vi "[RT] Finite Acq wRearm.vi"() -> ()   [LabVIEW 2015]
doc: "When a finite acquisition terminates, the FPGA automatically rearms itself for another acquisition. You simply need to call rwfm_Start.vi to perform another finite acquisition."
uses:
  <vilib>/NI/cRIO Wfm/ChannelConfig.ctl
  <vilib>/FPGAPlugInAG/sbRIO-9607/niLvFpga_Open_sbRIO-9607.vi
  <vilib>/rvi/interface/common/dynamic/niFpgaDynamicAddResources.vi
  <vilib>/FPGAPlugInAG/Dynamic/niLvFpga_Reset_Dynamic.vi
  <vilib>/FPGAPlugInAG/Dynamic/niLvFpga_Run_Dynamic.vi
  <vilib>/FPGAPlugInAG/Dynamic/niLvFpga_Close_Dynamic.vi
  <vilib>/rvi/interface/nirviOpenFPGA/nirviOpenFPGA.xnode
  FPGA Bitfiles/WaveformLibraryI_FPGATarget2_[FPGA]SARAcqMain_U+qOsuK4w1s.lvbitx
  FPGA/[FPGA] SAR Acq Main.vi
  <vilib>/rvi/interface/nirviMethod/nirviMethod.xnode
  <vilib>/rvi/interface/nirviCloseFPGA/nirviCloseFPGA.xnode
  IFw_Addon/RT/WaveformTask.lvclass
  <vilib>/NI/cRIO Wfm/cRIO Wfm.lvlib
panel:
  in  "Sample Rate":u32=51200
  in  "Channel Info":T1=[{"Channel Name"="Mod1/ai0", "Sensitivity mV_EU"=1000.0, "EU"="V", "dB Ref EU"=1.0}, {"Channel Name"="Mod1/ai1", "Sensitivity mV_EU"=1000.0, "EU"="V", "dB Ref EU"=1.0}, {"Channel Name"="Mod1/ai2", "Sensitivity mV_EU"=1000.0, "EU"="V", "dB Ref EU"=1.0}] caption="Channel Name      Scale [mV/EU]        EU           dB Ref [EU]" {"dB Ref EU" format="%#.2p"; "Sensitivity mV_EU" format="%.2f"}
  in  "Samps per Chan":i32=25600 caption="Samples per Channel"
  in  "stop":bool
  out "Waveform Graph":sgl[][](graph)
  in  "Snapshot":bool
  # "Sampling Info"
  # "Channel Info"
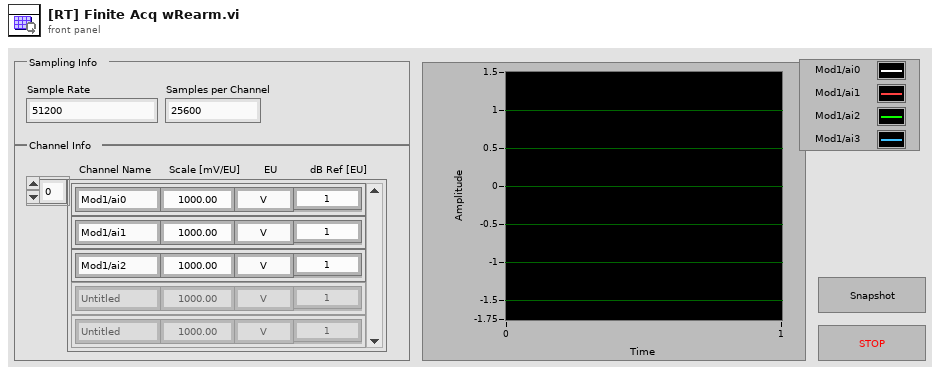
[diagram p1: front panel]
types:
  T1 = typedef "cRIO Wfm.lvlib/ChannelConfig.ctl" = cluster{"Channel Name":string, "Sensitivity mV_EU":dbl, "EU":string, "dB Ref EU":dbl}[]
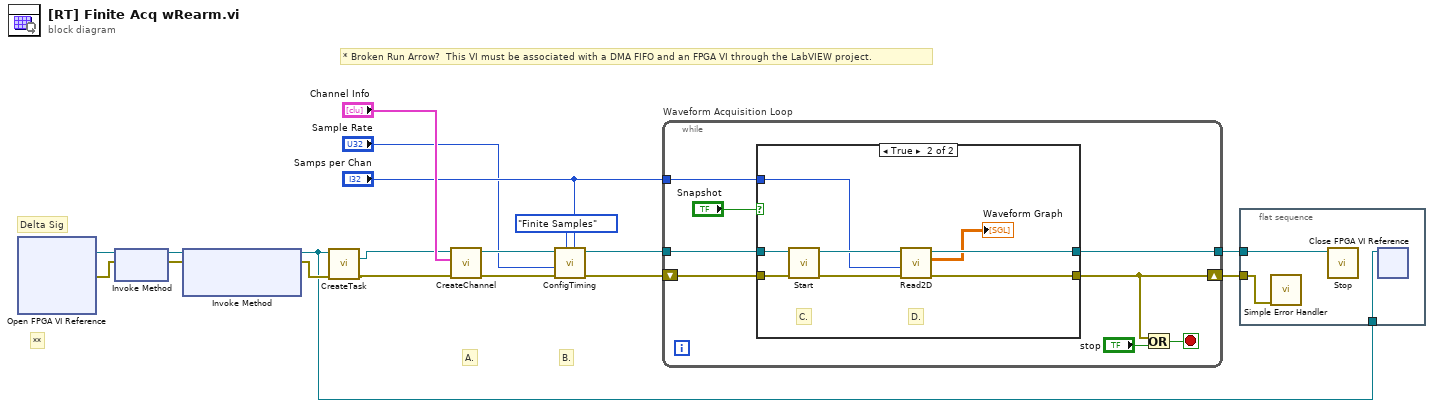
[diagram p0: block diagram]
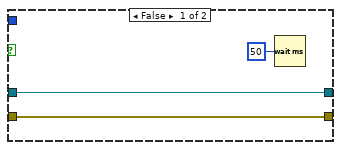
[diagram p2: hidden frame]
diagram:
  # "Delta Sig"
  # "**"
  # "* Broken Run Arrow?  This VI must be associated with a DMA FIFO and an FPGA VI through the LabVIEW project."
  # "B."
  # "A."
  n1 = xnode "Open FPGA VI Reference"() -> ("FPGA VI Reference Out"=w8:refnum<k20>, "error out"=w7:errorcluster)  [unwired: 2 in]
  n2 = xnode "Invoke Method"("FPGA VI Reference In"=w8, "error in"=w7) -> ("FPGA VI Reference Out"=w10:refnum<k20>, "error out"=w9:errorcluster)
  n3 = xnode "Invoke Method"("FPGA VI Reference In"=w10, "error in"=w9) -> ("FPGA VI Reference Out"=w2:refnum<k20>, "error out"=w6:errorcluster)  [unwired: 1 in]
  n4 = call "CreateTask.vi"("FPGA Ref in"=w2, "error in"=w6) -> ("Task out"=w5:refnum<class "WaveformTask.lvclass">, "error out"=w4:errorcluster)  [unwired: 11 in, 1 out]
  n5 = call "CreateChannel.vi"("error in"=w4, "Channel Info"="Channel Info", "task in"=w5) -> ("error out"=w14:errorcluster, "Task out"=w15:refnum<class "WaveformTask.lvclass">)  [unwired: 7 in]
  n6 = call "ConfigTiming.vi"("Samples per Channel"="Samps per Chan", "Sample Mode"=enum16{"Finite Samples", "Continuous Samples"}."Finite Samples", "error in (no error)"=w14, "Sample Rate"="Sample Rate", "Task in"=w15) -> ("error out"=w16:errorcluster, "Task out"=w17:refnum<class "WaveformTask.lvclass">)  [unwired: 4 in, 1 out]
  n7 = while "Waveform Acquisition Loop" {
    tunnel: w17 -> [w25]
    tunnel: [w24] -> w3
    tunnel: "Samps per Chan" -> [w20]
    shift-right: [w19] -> w1
    shift-left: w16 -> [w26]
    stop <- w22 stop-if-true
    n8 = case shown="True" "Snapshot" {
      tunnel: w26 -> [w28 w37]
      tunnel: w25 -> [w29 w36]
      tunnel: [w29 w35] -> w24
      tunnel: [w28 w34] -> w19
      tunnel: w20 -> [_ w30]
      frame False {
        n9 = Wait (ms)(milliseconds to wait=u32 50) -> ()  [unwired: 1 out]
      }
      frame True {
        # "C."
        # "D."
        n10 = call "Start.vi"("error in (no error)"=w37, "WaveformTask in"=w36) -> ("error out"=w33:errorcluster, "WaveformTask out"=w32:refnum<class "WaveformTask.lvclass">)  [unwired: 8 in]
        n11 = call "Read2D.vi"("error in"=w33, "Samps Read per Chan"=w30, "Task in"=w32) -> ("error out"=w34:errorcluster, "Data"=→"Waveform Graph":sgl[][], "Task out"=w35:refnum<class "WaveformTask.lvclass">)  [unwired: 5 in, 1 out]
      }
    }
    n12 = Or(x=w19, y="stop") -> (x .or. y?=w22:bool)
  }
  n13 = flat-sequence {
    tunnel: w3 -> [w40]
    tunnel: w2 -> [w39]
    tunnel: w1 -> [w38]
    frame #0 {
      n14 = call <vilib>:"Simple Error Handler.vi"("error in (no error)"=w38) -> ()  [unwired: 1 in, 8 out]
      n15 = call "Stop.vi"("WaveformTask in"=w40) -> ()  [unwired: 9 in, 2 out]
      n16 = xnode "Close FPGA VI Reference"("FPGA VI Reference In"=w39) -> ()  [unwired: 1 in, 1 out]
    }
  }
